vi "HFRR ADV v04 new software.vi"() -> ()   [LabVIEW 2025] (continued)
                n3603 = Set File Position(offset (in bytes) (0)=w4574, refnum=w4575, error in=w4576) -> (refnum out=w4567:refnum<file>, error out=w4566:errorcluster)  [unwired: 1 in]
                n3604 = Write to Binary File(file (use dialog)=w4567, data=w4572, error in=w4566, 5:FALSE ("prepend array or string size? (T)")) -> (error out=w4570:errorcluster)  [unwired: 2 in, 2 out]
                n3605 = flat-sequence {
                  tunnel: w4571 -> [w4586]
                  tunnel: w4570 -> [_]
                  frame #0 {
                    n3606 = call <vilib>:"Read Characters From File.vi"("file path (dialog if empty)"=w4586) -> ("character string"=→"Sensor Health JSON string":string)  [unwired: 5 in, 3 out]
                  }
                }
                "SinglePoint  2" <- w4572
              }
              frame #1 {
              }
              frame #2 {
                (unwired) "\"Stored\": true" ("string")
                n3607 = call <vilib>:"System Exec.vi"("run minimized? (F)"=TRUE, "wait until completion? (T)"=TRUE, "working directory"=path "C:/LAB-IQ-NXT", "command line"="C:\\LAB-IQ-NXT\\JPostH.bat") -> ("standard error"=→"Respose From Server 2":string, "standard output"=w4591:string)  [unwired: 4 in, 2 out]
                "standard output 2" <- w4591
                n3608 = Match Pattern(string=w4591, regular expression="JSONH Check String") -> (match substring=w4589:string, offset past match=w4588:i32)  [unwired: 1 in, 2 out]
                n3609 = Equal?(x=w4589, y="JSONH Check String") -> (x = y?=→"Upload \nConfirmed 2":bool)
              }
            }
            n3610 = Divide(x=w4431, y=3600.0 ("f")) -> (x/y=w4424:dbl)
            n3611 = local read "run time"() -> (w4481:string[])
            n3612 = Round To Nearest(number=w4424) -> (nearest integer value=w4423:dbl)
            n3613 = Number To Decimal String(number=w4423) -> (decimal integer string=w4422:string)  [unwired: 1 in]
            n3614 = Index Array(array="Sensor Information", index (col) #1=0 ("disabled index (col)"), index (col) #2=1 ("index (col)"), index (col) #3=2 ("index (col)"), index (col) #4=3 ("index (col)")) -> (element #1=→"Sensor name":string[], element #2=→"model num":string[], element #3=→"run time":string[], element #4=→"state":string[])  [unwired: 4 in]
            n3615 = Insert Into Array(array=w4481, index=1, new element #1=w4422, new element #2=w4422, new element #3=w4422, new element #4=w4422, new element #5=w4422, new element #6=w4422) -> (w4446:string[])
            "run" <- w4446
            n3616 = local read "out"() -> (w4428:string[])
            n3617 = local read "Sensor Information"() -> (w4448:string[][])
            n3618 = Replace Array Subset(array=w4448, new element #1=w4446, index (col) #1=2 ("disabled index (col)"), new element #2=w4428, index (col) #2=3 ("index (col)")) -> (w4447:string[][])  [unwired: 2 in]
            n3619 = local write "Sensor Information"(w4447) -> ()
          }
        }
        n3620 = case shown="True" w4395 {
          frame False {
          }
          frame True {
            n3621 = Equal?(x="FLAG", y=0.0) -> (x = y?=w4412:bool)
            n3622 = case shown="False" w4412 {
              frame False {
                n3623 = Get Date/Time In Seconds() -> (seconds since 1Jan1904=w4418:timestamp)
                n3624 = local read "START 2"() -> (w4416:dbl)
                n3625 = To Double Precision Float(number=w4418) -> (double precision float=w4417:dbl)
                n3626 = Subtract(x=w4417, y=w4416) -> (x-y=→"SENSOR TIME  2":dbl)
              }
              frame True {
                n3627 = Get Date/Time In Seconds() -> (seconds since 1Jan1904=w4420:timestamp)
                n3628 = To Double Precision Float(number=w4420) -> (double precision float=→"START 2":dbl)
                n3629 = local write "FLAG"(100.0 ("FLAG")) -> ()
              }
            }
          }
        }
        n3630 = disable-structure shown="Disabled" {
          disable-tunnel: w4398 -> [w4407 _]
          disable-tunnel: [w4406 _] -> w4397
          frame Disabled {
            n3631 = local read "Json St Flg"() -> (w4405:bool)
            n3632 = case shown="True" w4405 {
              tunnel: w4407 -> [w4408 w4410]
              tunnel: [w4408 w4409] -> w4406
              frame False {
              }
              frame True {
                n3633 = Increment(x=w4410) -> (x+1=w4409:dbl)
                "T cycle" <- w4409
                n3634 = local write "Json St Flg"(FALSE ("Json St Flg")) -> ()
              }
            }
          }
          frame Enabled {
          }
        }
        n3635 = local read "Quit"() -> (w4392:bool)
      }
    }
    frame Enabled {
    }
  }
  n3636 = stacked-sequence {
    tunnel: [w4790] -> w38
    frame #0 {
      w4790 = FALSE ("Upload \nConfirmed")
      n3637 = local write "Upload \nConfirmed"(w4790) -> ()
      n3638 = local write "St Str"("") -> ()
    }
  }
  n3639 = disable-structure shown="Disabled" {
    disable-tunnel: w38 -> [w4791 _]
    frame Disabled {
      n3640 = case shown="True" {
        selector: _ -> [_ _]
        tunnel: w4791 -> [_ w4792]
        frame False {
        }
        frame True {
          n3641 = while {
            tunnel: [w4798] -> _
            tunnel: w4792 -> [_]
            i -> [w4798]
            stop <- w4793 stop-if-true
            n3642 = local read "Json End Flg"() -> (w4797:bool)
            n3643 = Wait (ms)(milliseconds to wait=u32 20 ("Refresh Rate (ms)")) -> ()  [unwired: 1 out]
            n3644 = local read "refresh flag"() -> (w4794:bool)
            n3645 = local read "RUN"() -> (w4795:bool)
            n3646 = And(x=w4795, y=w4794) -> (x .and. y?=w4796:bool)
            n3647 = Or(x=w4796, y=w4797) -> (x .or. y?=w4799:bool)
            "AR Led" <- w4799
            n3648 = case shown="True" w4799 {
              frame False {
              }
              frame True {
                w4816 = "\",\""
                n3649 = local read "UUID"() -> (w4814:string)
                n3650 = local write "refresh flag"(FALSE ("refresh flag")) -> ()
                n3651 = local read "time"() -> (w4803:dbl)
                n3652 = Multiply(x=w4803, y=60.0) -> (x*y=w4802:dbl)
                n3653 = Concatenate Strings("UUID\" : \"", w4814, "\"}") -> (w4817:string)
                n3654 = Number To Fractional String(number=w4802, width (-)=i16 10, precision (6)=i16 4) -> (F-format string=w4831:string)  [unwired: 1 in]
                n3655 = Concatenate Strings("{", "\"Time\":\"", w4831, w4816) -> (w4826:string)
                n3656 = stacked-sequence {
                  tunnel: w4816 -> [w4879 w4887 w4894 w4902 w4910 w4919 w4926]
                  tunnel: [w4880 _ _ _ _ _ _] -> w4830
                  tunnel: [_ w4888 _ _ _ _ _] -> w4829
                  tunnel: [_ _ w4895 _ _ _ _] -> w4828
                  tunnel: [_ _ _ w4904 _ _ _] -> w4827
                  tunnel: w4817 -> [_ _ _ _ _ _ w4937]
                  tunnel: [_ _ _ _ _ _ w4936] -> w4813
                  tunnel: [_ _ _ _ _ w4916 _] -> w4812
                  tunnel: [_ _ _ _ w4909 _ _] -> w4811
                  frame #0 {
                    n3657 = local read "NORMAL LOAD"() -> (w4878:dbl)
                    n3658 = Number To Fractional String(number=w4878, width (-)=i16 10, precision (6)=i16 4) -> (F-format string=w4881:string)  [unwired: 1 in]
                    n3659 = Concatenate Strings("NormalLoad\":\"", w4881, w4879) -> (w4880:string)
                  }
                  frame #1 {
                    n3660 = local read "Temp"() -> (w4886:dbl)
                    n3661 = Number To Fractional String(number=w4886, width (-)=i16 10, precision (6)=i16 4) -> (F-format string=w4889:string)  [unwired: 1 in]
                    n3662 = Concatenate Strings("Temperature\":\"", w4889, w4887) -> (w4888:string)
                  }
                  frame #2 {
                    n3663 = local read "cof"() -> (w4892:dbl)
                    n3664 = Number To Fractional String(number=w4892, width (-)=i16 10, precision (6)=i16 4) -> (F-format string=w4896:string)  [unwired: 1 in]
                    n3665 = Concatenate Strings("FrictionalForce\":\"", w4896, w4894) -> (w4895:string)
                  }
                  frame #3 {
                    n3666 = local read "Set Hz"() -> (w4900:dbl)
                    n3667 = Multiply(x=w4900, y=60.0) -> (x*y=w4899:dbl)
                    n3668 = Number To Fractional String(number=w4899, width (-)=i16 10, precision (6)=i16 4) -> (F-format string=w4905:string)  [unwired: 1 in]
                    n3669 = Concatenate Strings("Speed\":\"", w4905, w4902) -> (w4904:string)
                  }
                  frame #4 {
                    n3670 = local read item#-1() -> (w4908)
                    n3671 = Number To Fractional String(number=w4908, width (-)=i16 10, precision (6)=i16 4) -> (F-format string=w4912:string)  [unwired: 1 in]
                    n3672 = Concatenate Strings("LinearDeformation\":\"", w4912, w4910) -> (w4909:string)
                  }
                  frame #5 {
                    n3673 = local read "AIR TEMP"() -> (w4915:dbl)
                    n3674 = local read "Json St Flg"() -> (w4917:bool)
                    n3675 = local read "Json End Flg"() -> (w4918:bool)
                    n3676 = Number To Fractional String(number=w4915, width (-)=i16 10, precision (6)=i16 4) -> (F-format string=w4921:string)  [unwired: 1 in]
                    n3677 = Concatenate Strings("Vibration\":\"", w4921, w4919) -> (w4916:string)
                    n3678 = And(x=w4917, y=w4918) -> ()  [unwired: 1 out]
                  }
                  frame #6 {
                    n3679 = local read "Json End Flg"() -> (w4925:bool)
                    n3680 = Get Date/Time In Seconds() -> (seconds since 1Jan1904=w4933:timestamp)
                    n3681 = local read "Json St Flg"() -> (w4924:bool)
                    n3682 = To Double Precision Float(number=w4933) -> (double precision float=w4932:dbl)
                    n3683 = Subtract(x=w4932, y=2082844800.0) -> (x-y=w4930:dbl)
                    n3684 = Number To Fractional String(number=w4930, width (-)=i16 12, precision (6)=i16 0) -> (F-format string=w4927:string)  [unwired: 1 in]
                    n3685 = case shown="True" w4925 {
                      tunnel: ["" w4940] -> w4934
                      tunnel: w4927 -> [_ w4941]
                      tunnel: w4926 -> [_ w4939]
                      frame False {
                      }
                      frame True {
                        n3686 = local write "Json End Flg"(FALSE ("Json St Flg")) -> ()
                        n3687 = Concatenate Strings("End\": \"", w4941, w4939) -> (w4940:string)
                      }
                    }
                    n3688 = case shown="True" w4924 {
                      tunnel: [w4944 w4947] -> w4935
                      tunnel: w4927 -> [_ w4948]
                      tunnel: w4926 -> [_ w4945]
                      frame False {
                        n3689 = local read "St Str"() -> (w4944:string)
                      }
                      frame True {
                        n3690 = Concatenate Strings("Start\":\"", w4948, w4945) -> (w4947:string)
                        "St Str" <- w4947
                        n3691 = local write "Json St Flg"(FALSE ("Json St Flg")) -> ()
                      }
                    }
                    n3692 = Concatenate Strings(w4935, w4934, w4937) -> (w4936:string)
                  }
                }
                n3693 = local read "FILE"() -> (w4805:string)
                n3694 = Concatenate Strings("\",\"OperatorID\":\"" ("string"), "Operator ID") -> (w4808:string)
                n3695 = Concatenate Strings("\",\"DatasetTitle\":\"" ("string"), w4805) -> (w4807:string)
                n3696 = Concatenate Strings("\",\"SerialNumber\":\"" ("string"), "Serial No") -> (w4837:string)
                n3697 = Concatenate Strings("\",\"ModelNumber\":\"" ("string"), "Model No") -> (w4836:string)
                n3698 = Concatenate Strings(w4837, w4836) -> (w4819:string)
                n3699 = Concatenate Strings("{\"SecretKey\":\"", "Secret Key", w4819, w4808, w4807, "\",\"Samples\":[") -> (w4824:string)
                n3700 = Concatenate Strings(w4826, w4830, w4829, w4828, w4827, w4811, w4812, w4813) -> (w4825:string)
                n3701 = Concatenate Strings(w4824, w4825, "]}") -> (w4823:string)
                n3702 = stacked-sequence {
                  tunnel: w4823 -> [w4852 _ _]
                  tunnel: [_ _ w4869] -> _
                  frame #0 {
                    (unwired) FALSE ("convert eol (F)")
                    w4854 = enum16{"start", "end", "current"}."start" ("pos mode (0:2)")
                    n3703 = Path To String(path="Path") -> (string=w4860:string)
                    n3704 = Concatenate Strings(w4860, "\\", "Data File Name") -> (w4862:string)
                    n3705 = local write "standard output"(" ") -> ()
                    n3706 = String To Path(string=w4862) -> (path=w4851:path)
                    n3707 = call <vilib>:"Open_Create_Replace File.vi"("advisory dialog? (display:T)"=FALSE, "function (open:0)"=T25."create or replace", "file path"=w4851) -> ("error out"=w4865:errorcluster, "refnum"=w4864:refnum<file>)  [unwired: 5 in, 2 out]
                    n3708 = Set File Position(refnum=w4864, from (0:start)=w4854, error in=w4865) -> (refnum out=w4845:refnum<file>, error out=w4844:errorcluster)  [unwired: 1 in]
                    n3709 = Write to Binary File(file (use dialog)=w4845, data=" ", error in=w4844, 5:FALSE ("prepend array or string size? (T)")) -> (refnum out=w4855:refnum<file>, error out=w4856:errorcluster)  [unwired: 2 in, 1 out]
                    n3710 = Set File Position(offset (in bytes) (0)=w4854, refnum=w4855, error in=w4856) -> (refnum out=w4848:refnum<file>, error out=w4847:errorcluster)  [unwired: 1 in]
                    n3711 = Write to Binary File(file (use dialog)=w4848, data=w4852, error in=w4847, 5:FALSE ("prepend array or string size? (T)")) -> (error out=w4850:errorcluster)  [unwired: 2 in, 2 out]
                    n3712 = flat-sequence {
                      tunnel: w4851 -> [w4867]
                      tunnel: w4850 -> [_]
                      frame #0 {
                        n3713 = call <vilib>:"Read Characters From File.vi"("file path (dialog if empty)"=w4867) -> ("character string"=→"JSON string":string)  [unwired: 5 in, 3 out]
                      }
                    }
                    "SinglePoint" <- w4852
                  }
                  frame #1 {
                  }
                  frame #2 {
                    (unwired) "\"Stored\": true" ("string")
                    n3714 = call <vilib>:"System Exec.vi"("run minimized? (F)"=TRUE, "wait until completion? (T)"=TRUE, "working directory"=path "C:/LAB-IQ-NXT", "command line"="C:\\LAB-IQ-NXT\\JPost.bat") -> ("standard error"=→"Respose From Server":string, "standard output"=w4872:string)  [unwired: 4 in, 2 out]
                    "standard output" <- w4872
                    n3715 = Match Pattern(string=w4872, regular expression="JSON Check String") -> (match substring=w4870:string, offset past match=w4869:i32)  [unwired: 1 in, 2 out]
                    n3716 = Equal?(x=w4870, y="JSON Check String") -> (x = y?=→"Upload \nConfirmed":bool)
                  }
                }
              }
            }
            n3717 = local read "Quit"() -> (w4793:bool)
          }
        }
      }
    }
    frame Enabled {
    }
  }
  n3718 = disable-structure shown="Disabled" {
    disable-tunnel: _ -> [w4955 _]
    frame Disabled {
      n3719 = while {
        shift-right: [w4963] -> w4951
        shift-left: _ -> [w4964]
        shift-right: [w4961] -> w4952
        shift-left: errorcluster {"status"=TRUE, "code"=0, "source"="Init"} ("error out") -> [w4962]
        shift-right: [w4959] -> _
        shift-left: "" -> [w4960]
        tunnel: [w4957] -> _
        tunnel: w4955 -> [_]
        i -> [w4957]
        stop <- w4956 stop-if-true
        n3720 = flat-sequence {
          tunnel: [w4965] -> w4958
          frame #0 {
            n3721 = Wait (ms)(milliseconds to wait=10.0 ("Delay")) -> (millisecond timer value=w4965:u32)
          }
        }
        n3722 = case shown="No Error" w4962 {
          selector: w4962 -> [w4995 w5114]
          tunnel: [w4978 w5116] -> w4963
          tunnel: [w4977 w5115] -> w4961
          tunnel: w4964 -> [w4996 w5108]
          tunnel: w4960 -> [w4976 w5107]
          tunnel: [w4975 w5107] -> w4959
          tunnel: w4958 -> [_ _]
          frame No Error {
            n3723 = Concatenate Strings("\r", "\n") -> (w4987:string)  [unwired: 1 in]
            n3724 = case shown="True" w4988 {
              tunnel: w4996 -> [w5020 w5027]
              tunnel: w4995 -> [w5019 w5026]
              tunnel: [w5020 w5025] -> w4994
              tunnel: [w5019 w5024] -> w4974
              tunnel: w4987 -> [_ w5023]
              frame False {
              }
              frame True {
                n3725 = VISA Write(VISA resource name=w5027, write buffer=w5023, error in (no error)=w5026) -> (VISA resource name out=w5025:refnum<visa-resource-name>, error out=w5024:errorcluster)  [unwired: 1 out]
                n3726 = local write "Read String"("") -> ()
                n3727 = local write item#-1(FALSE) -> ()
              }
            }
            n3728 = property class="Instr"(reference=w4994, error in=w4974) -> (reference out=w4993:refnum<visa-resource-name>, error out=w4992:errorcluster, "Serial Settings:Number of Bytes at Serial Port"=w4991:u32)
            n3729 = Greater?(x=w4991, y=u32 100) -> (0:w4989:bool)
            n3730 = case shown="True" w4989 {
              tunnel: w4993 -> [w5030 w5054]
              tunnel: w4992 -> [w5029 w5053]
              tunnel: w4991 -> [_ w5052]
              tunnel: [w5030 w5051] -> w4980
              tunnel: [w5029 w5050] -> w4979
              tunnel: w4976 -> [w5028 w5049]
              tunnel: [w5028 ""] -> w4975
              frame False {
              }
              frame True {
                w5039 = u32 6 ("y")
                # "Page 84 of \nmanual"
                n3731 = VISA Read(VISA resource name=w5054, byte count=w5052, error in (no error)=w5053) -> (VISA resource name out=w5051:refnum<visa-resource-name>, read buffer=w5047:string, error out=w5050:errorcluster)  [unwired: 1 out]
                n3732 = while {
                  tunnel: w5047 -> [w5103]
                  tunnel: [w5099] -> w5041 mode=indexing
                  tunnel: [w5093] -> w5045 mode=indexing
                  tunnel: [w5091] -> _
                  i -> [w5091]
                  stop <- w5096 stop-if-true
                  n3733 = String Subset(string=w5103, offset (0)=w5091) -> (substring=w5098:string)  [unwired: 1 in]
                  n3734 = String To Byte Array(string=w5098) -> (unsigned byte array=w5102:u8[])
                  n3735 = String Length(string=w5098) -> (length=w5097:i32)
                  n3736 = Index Array(array=w5102) -> (element=w5101:u8)  [unwired: 1 in]
                  n3737 = Equal To 0?(x=w5097) -> (x = 0?=w5096:bool)
                  n3738 = Number To Boolean Array(number=w5101) -> (Boolean array=w5095:bool[])
                  n3739 = Reverse 1D Array(array=w5095) -> (reversed array=w5094:bool[])
                  n3740 = And(x=w5095, y=bool[] [FALSE, FALSE, FALSE, FALSE, FALSE, FALSE, TRUE, TRUE] ("Boolean array")) -> (x .and. y?=w5099:bool[])
                  n3741 = And(x=w5094, y=bool[] [FALSE, FALSE, TRUE, TRUE, TRUE, TRUE, TRUE, TRUE] ("Boolean array")) -> (x .and. y?=w5093:bool[])
                }
                n3742 = Concatenate Strings(w5049, w5047) -> (→"Read String":string)
                n3743 = while {
                  tunnel: w5041 -> [w5090] mode=indexing
                  tunnel: [w5086] -> w5044
                  i -> [w5086]
                  stop <- w5087 stop-if-true
                  n3744 = Search 1D Array(1D array=w5090, element=TRUE) -> (index of element=w5088:i32)  [unwired: 1 in]
                  n3745 = Less Than 0?(x=w5088) -> (x < 0?=w5087:bool)
                }
                n3746 = Delete From Array(array=w5045, length=w5044, index (row)=0) -> (array with subset deleted=w5040:bool[][])  [unwired: 1 in, 1 out]
                n3747 = Array Size(array=w5040) -> (size(s)=w5042:i32[])
                n3748 = Index Array(array=w5042) -> (element=w5034:i32)  [unwired: 1 in]
                n3749 = Greater?(x=w5034, y=w5039) -> (0:w5037:bool)
                n3750 = Subtract(x=w5034, y=w5039) -> (x-y=w5038:u32)
                n3751 = Select(t=w5038, s=w5037, f=u32 0) -> (s? t:f=w5035:u32)
                n3752 = while {
                  tunnel: w5040 -> [w5073]
                  tunnel: [w5075] -> w5033 mode=indexing
                  tunnel: w5035 -> [w5057]
                  i -> [w5074]
                  stop <- w5072 stop-if-true
                  w5064 = 6 ("index")
                  w5063 = 2 ("length")
                  # "Page 65 of \nmanual"
                  n3753 = Multiply(x=u32 3 ("y"), y=w5074) -> (x*y=w5071:u32)
                  n3754 = Divide(x=u32 102 ("y"), y=u32 65520) -> (x/y=w5081:dbl)
                  n3755 = Greater Or Equal?(x=w5071, y=w5057) -> (x >= y?=w5072:bool)
                  n3756 = Index Array(array=w5073, index (row) #1=w5071) -> (element #1=w5069:bool[], element #2=w5068:bool[], element #3=w5067:bool[])  [unwired: 5 in]
                  n3757 = Reverse 1D Array(array=w5069) -> (reversed array=w5062:bool[])
                  n3758 = Reverse 1D Array(array=w5068) -> (reversed array=w5066:bool[])
                  n3759 = Reverse 1D Array(array=w5067) -> (reversed array=w5065:bool[])
                  n3760 = Delete From Array(array=w5062, length=w5063, index=w5064) -> (array with subset deleted=w5058:bool[])  [unwired: 1 out]
                  n3761 = Delete From Array(array=w5066, length=w5063, index=w5064) -> (array with subset deleted=w5059:bool[])  [unwired: 1 out]
                  n3762 = Delete From Array(array=w5065, length=w5063, index=w5064) -> (array with subset deleted=w5060:bool[])  [unwired: 1 out]
                  n3763 = Insert Into Array(array=bool[] [] ("Boolean array"), new element #1=w5058, new element #2=w5059, new element #3=w5060) -> (w5061:bool[])  [unwired: 1 in]
                  n3764 = Boolean Array To Number(Boolean array=w5061) -> (number=w5070:u32)
                  n3765 = Multiply(x=w5081, y=w5070) -> (x*y=w5080:dbl)
                  n3766 = Decrement(x=w5080) -> (x-1=w5079:dbl)
                  n3767 = Divide(x=w5079, y=u32 100) -> (x/y=w5077:dbl)
                  n3768 = Multiply(x=w5077, y=u32 10) -> (x*y=w5075:dbl)
                }
                n3769 = Delete From Array(array=w5033) -> (array with subset deleted=w5032:dbl[])  [unwired: 2 in, 1 out]
                "Waveform Graph 5" <- w5032
                "Waveform Chart 3" <- w5032
                n3770 = call-poly <vilib>:"Mean.vi"("X"=w5032) -> ("mean"=w5031:dbl)  [unwired: 1 out]
                n3771 = case shown="True" {
                  selector: _ -> [_ _]
                  tunnel: w5031 -> [_ w5056]
                  frame False {
                  }
                  frame True {
                    n3772 = local write item#-1(FALSE ("Zero 4")) -> ()
                    "z_measure" <- w5056
                  }
                }
              }
            }
            n3773 = local read item#-1() -> (w4971)
            n3774 = local read item#-1() -> (w4970)
            n3775 = local read item#-1() -> (w4972)
            n3776 = local read item#-1() -> (w4969)
            n3777 = case shown="True" w4967 {
              tunnel: w4971 -> [_ w4999]
              tunnel: w4972 -> [_ w4998]
              frame False {
              }
              frame True {
                n3778 = Build Array(w4999, w4998) -> (w4997:void[])
                n3779 = local read item#-1() -> (w5002)
                n3780 = Build Array (concatenate)(w5002, w4997) -> (w5000:void[])
                n3781 = local write item#-1(w5000) -> ()
                n3782 = local write item#-1(FALSE ("Boolean 8")) -> ()
              }
            }
            n3783 = call "Build XY Graph"("Enable"=w4969, "Reset"=w4970, "Y Input"=w4972, "X Input"=w4971) -> ("XY Graph"=w4968:cluster{"Y":dbl[], "Y":dbl[]}[])  [unwired: 6 in, 1 out]
            n3784 = case shown="True" {
              selector: _ -> [_ _]
              frame False {
              }
              frame True {
                n3785 = local read item#-1() -> (w5003)
                n3786 = Index Array(array=w5003, index (col) #1=0 ("disabled index (col)"), index (col) #2=1 ("index (col)")) -> (element #1=w5005, element #2=w5004)  [unwired: 2 in]
                n3787 = call <vilib>:"Linear Fit.vi"("Y"=w5005, "X"=w5004) -> ()  [unwired: 9 in, 5 out]
                n3788 = local write item#-1(FALSE ("Boolean 9")) -> ()
              }
            }
            n3789 = case shown="True" {
              selector: _ -> [_ _]
              frame False {
              }
              frame True {
                n3790 = local write item#-1(dbl[][] [] ("Captured Values")) -> ()
                n3791 = local write item#-1(FALSE ("Boolean 7")) -> ()
              }
            }
            n3792 = Concatenate Strings("\r", "\n") -> (w4982:string, w4981:string)
            n3793 = case shown="True" w4973 {
              tunnel: w4980 -> [w5012 w5018]
              tunnel: w4979 -> [w5011 w5017]
              tunnel: [w5012 w5016] -> w4978
              tunnel: [w5011 w5015] -> w4977
              tunnel: w4982 -> [_ w5014]
              frame False {
              }
              frame True {
                n3794 = VISA Write(VISA resource name=w5018, write buffer=w5014, error in (no error)=w5017) -> (VISA resource name out=w5016:refnum<visa-resource-name>, error out=w5015:errorcluster)  [unwired: 1 out]
                n3795 = local write item#-1(FALSE ("WRITE")) -> ()
              }
            }
          }
          frame Error {
            w5106 = u16 10 items=["1.0"=10, "1.5"=15, "2.0"=20] ("stop bits (10: 1 bit)")
            n3796 = Wait (ms)(milliseconds to wait=u32 20) -> ()  [unwired: 1 out]
            n3797 = VISA Close(VISA resource name=w5108, error in (no error)=w5114) -> (error out=w5113:errorcluster)
            n3798 = call <vilib>:"Clear Errors.vi"("error in (no error)"=w5113) -> ("error out"=w5112:errorcluster)  [unwired: 5 in, 1 out]
            n3799 = call-poly "VISA Configure Serial Port"("timeout (10sec)"=u32 200, "Enable Termination\nChar (T)"=TRUE ("Enable Termination\nChar (T)"), "baud rate (9600)"=u32 921600, "error in (no error)"=w5112, "stop bits (10: 1 bit)"=w5106) -> ("VISA resource name"=w5104:refnum<visa-resource-name>, "VISA resource name out"=w5116:refnum<visa-resource-name>, "error out"=w5115:errorcluster)  [unwired: 8 in]
          }
        }
        n3800 = local read "Quit"() -> (w4956:bool)
      }
      n3801 = VISA Close(VISA resource name=w4951, error in (no error)=w4952) -> (error out=w4950:errorcluster)
      n3802 = call <vilib>:"Clear Errors.vi"("error in (no error)"=w4950) -> ()  [unwired: 5 in, 2 out]
    }
    frame Enabled {
    }
  }
  n3803 = disable-structure shown="Disabled" {
    disable-tunnel: _ -> [w5121 _]
    frame Disabled {
      n3804 = while {
        tunnel: [w5128] -> _
        shift-right: [w5125] -> w5118
        shift-left: _ -> [w5127]
        shift-right: [w5126] -> w5119
        shift-left: errorcluster {"status"=TRUE, "code"=0, "source"="Init"} ("error out") -> [w5124]
        tunnel: w5121 -> [_]
        i -> [w5128]
        stop <- w5122 stop-if-true
        n3805 = flat-sequence {
          tunnel: w5124 -> [w5219]
          tunnel: [w5219] -> w5123
          frame #0 {
            n3806 = Wait (ms)(milliseconds to wait=u32 50) -> ()  [unwired: 1 out]
          }
        }
        n3807 = case shown="No Error" w5123 {
          selector: w5123 -> [w5169 w5212]
          tunnel: w5127 -> [w5168 w5211]
          tunnel: [w5135 w5202] -> w5126
          tunnel: [w5136 w5210] -> w5125
          frame No Error {
            w5162 = T26 {"Mode"=enum."RTU", "Slave Address"=1} ("Serial Parameters")
            n3808 = call-poly <vilib>:"MB Serial Master Query (poly).vi"("VISA resource name"=w5168, "Starting Address"=i16 1000, "Quantity"=u16 1, "Timeout"=u32 1000, "error in"=w5169, "Serial Parameters"=w5162) -> ("VISA resource name out"=w5163:refnum<visa-resource-name>, "Input Registers"=w5165:u16[], "error out"=w5161:errorcluster)  [unwired: 10 in, 1 out]
            n3809 = Random Number (0-1)() -> (number: 0 to 1=w5150:dbl)
            n3810 = Index Array(array=w5165, index=0) -> (element=w5160:u16)
            n3811 = Subtract(x=w5150, y=0.5) -> (x-y=w5149:dbl)
            n3812 = Divide(x=w5160, y=10 ("index")) -> (x/y=w5154:dbl)
            n3813 = Multiply(x=w5149, y=0.5) -> (x*y=w5148:dbl)
            n3814 = Add(x=w5154, y=w5148) -> (x+y=w5153:dbl)
            n3815 = local read "Amb temp"() -> (w5137:dbl)
            n3816 = Multiply(x=w5153, y=0.2) -> (x*y=w5157:dbl)
            n3817 = Multiply(x=w5137, y=0.8) -> (x*y=w5155:dbl)
            n3818 = Add(x=w5157, y=w5155) -> (x+y=w5138:dbl)
            n3819 = local read "set temp old"() -> (w5132:dbl)
            n3820 = local write "Amb temp"(w5138) -> ()
            n3821 = Select(t="SetTemp 2", s="Heater", f=100.0) -> (s? t:f=w5133:dbl)
            n3822 = Not Equal?(x=w5133, y=w5132) -> (x != y?=w5131:bool)
            n3823 = case shown="True" w5131 {
              tunnel: w5163 -> [w5197 w5199]
              tunnel: [w5196 w5199] -> w5143
              tunnel: w5161 -> [w5195 w5198]
              tunnel: [w5194 w5198] -> w5141
              tunnel: w5133 -> [w5189 _]
              tunnel: w5162 -> [w5191 w5200]
              tunnel: [w5191 w5200] -> w5144
              frame True {
                n3824 = Multiply(x=w5189, y=10 ("index")) -> (x*y=w5188:dbl)
                n3825 = call-poly <vilib>:"MB Serial Master Query (poly).vi"("VISA resource name"=w5197, "Address"=u16 0, "Holding Register"=w5188, "Timeout"=u32 1000, "error in"=w5195, "Serial Parameters"=w5191) -> ("VISA resource name out"=w5196:refnum<visa-resource-name>, "error out"=w5194:errorcluster)  [unwired: 11 in, 1 out]
                "set temp old" <- w5189
              }
              frame False {
              }
            }
            n3826 = flat-sequence {
              tunnel: [w5170] -> _
              tunnel: [w5170] -> w5140
              tunnel: w5141 -> [w5170]
              frame #0 {
                n3827 = Wait (ms)(milliseconds to wait=u32 100) -> ()  [unwired: 1 out]
              }
            }
            n3828 = call "Elapsed Time12"("Time Target (s)"=2.0, "Auto Reset"=TRUE) -> ("Time has Elapsed"=w5145:bool)  [unwired: 10 in, 7 out]
            n3829 = case shown="True" w5145 {
              tunnel: w5144 -> [w5174 w5187]
              tunnel: [w5174 w5187] -> _
              tunnel: [w5173 w5185] -> w5136
              tunnel: w5143 -> [w5173 w5186]
              tunnel: [w5172 w5183] -> w5135
              tunnel: w5140 -> [w5172 w5184]
              frame False {
              }
              frame True {
                n3830 = call-poly <vilib>:"MB Serial Master Query (poly).vi"("VISA resource name"=w5186, "Starting Address"=i16 1003 ("Addr"), "Quantity"=u16 1, "Timeout"=u32 1000, "error in"=w5184, "Serial Parameters"=w5187) -> ("VISA resource name out"=w5185:refnum<visa-resource-name>, "Input Registers"=w5180:u16[], "error out"=w5183:errorcluster)  [unwired: 10 in, 1 out]
                n3831 = Index Array(array=w5180, index=0) -> (element=w5179:u16)
                n3832 = Divide(x=w5179, y=u16 10) -> (x/y=w5175:dbl)
                n3833 = local write "set temp old"(w5175) -> ()
                n3834 = local write "SetTemp"(w5175) -> ()
              }
            }
            "Error Code" <- w5135
            n3835 = Unbundle(w5135) -> ("status"=→"TK4 status":bool)  [unwired: 2 out]
            "SetTemp" <- "SetTemp 2"
          }
          frame Error {
            w5214 = u16 0 items=["None", "Odd", "Even", "Mark", "Space"] ("Parity")
            w5215 = u16 0 items=["None", "XON/XOFF", "RTS/CTS", "XON/XOFF & RTS/CTS", "DTR/DSR", "XON/XOFF & DTR/DSR"] ("Flow Control")
            n3836 = VISA Clear(VISA resource name=w5211, error in (no error)=w5212) -> (VISA resource name out=w5205:refnum<visa-resource-name>, error out=w5203:errorcluster)
            n3837 = VISA Close(VISA resource name=w5205, error in (no error)=w5203) -> (error out=w5204:errorcluster)
            n3838 = call <vilib>:"Clear Errors.vi"("error in (no error)"=w5204) -> ("error out"=w5213:errorcluster)  [unwired: 5 in, 1 out]
            n3839 = Unbundle By Name(T26 {"Mode"=enum."RTU", "Slave Address"=1} ("input cluster")) -> ("Mode"=w5216:enum16{"RTU", "ASCII"})
            n3840 = call <vilib>:"MB Serial Init.vi"("Timeout"=u32 100, "Flow Control"=w5215, "Mode"=w5216, "error in (no error)"=w5213, "Parity"=w5214, "Baud Rate"=u32 9600, "VISA resource name"="Lubrication System COM Port :") -> ("error out"=w5202:errorcluster, "VISA resource name out"=w5210:refnum<visa-resource-name>)  [unwired: 3 in]
            n3841 = local write "set temp old"(0.0 ("set temp old")) -> ()
            n3842 = Unbundle(w5202) -> ("status"=w5201:bool)  [unwired: 2 out]
            n3843 = case shown="True" w5201 {
              selector: w5201 -> [_ w5218]
              frame False {
              }
              frame True {
                n3844 = local write "TK4 status"(w5218) -> ()
              }
            }
          }
        }
        n3845 = local read "Quit"() -> (w5122:bool)
      }
      n3846 = VISA Close(VISA resource name=w5118, error in (no error)=w5119) -> (error out=w5117:errorcluster)
      n3847 = call <vilib>:"Clear Errors.vi"("error in (no error)"=w5117) -> ()  [unwired: 5 in, 2 out]
    }
    frame Enabled {
    }
  }
